vi "CRYMain Menu Process.vi"(3 "Sub Menu String":string, 4 "Menu String":string, 5 "nData":i32) -> (1 "sData_Out":string)   [LabVIEW 2013]
doc: "This is a subVI for the Block Menu Demo.vi. It is used as a pop-up subVI that displays a progress indicator."
uses:
  CRYProject/CRYProject Editor Global.vi
  CRYMainGlobal.vi
  DataView/VIEW/CRYView Global.vi
  DataView/VIEW/CRYNew View Global.vi
  CRYStepSetup/CRYStepSetup Global.vi
  CRYSystem/Task Sequence/CRYProject Run Control Global.vi
  SubVI/CRYMain Sub Window Global.vi
  CRYSystem/Data/CRYData & result stacks global.vi
  CRYSystem/Program/CRYRef nums global.vi
  CRYSystem/Misc/SubVI/CRYMisc vis settings global.vi
  <vilib>/Platform/browser.llb/Open URL in Default Browser (string).vi
  <vilib>/Platform/browser.llb/Open URL in Default Browser (path).vi
  <vilib>/Utility/miscctls.llb/LVRectTypeDef.ctl
panel:
  out "sData":string
  in  "pVIRef 2":refnum<vi>
  in  "pVIRef":refnum<vi>
  # "Main Menu Process"
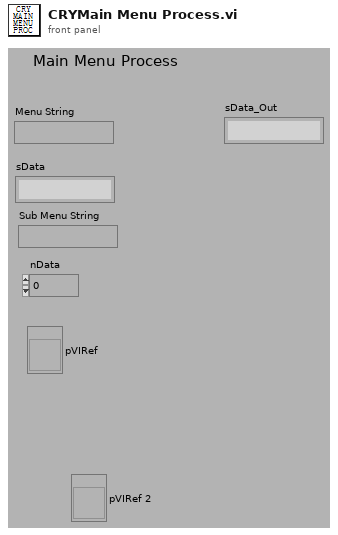
[diagram p1: front panel]
types:
  T1 = cluster{"EventName":string, "Arg1":string, "Numeric":u16, "Numeric 2":u16, "AddSteps ":refnum<vi>, "Arg1 2":string, "Arg1 3":string, "Boolean":bool}
  T2 = enum32{"Invalid", "Standard", "Closed", "Hidden", "Minimized", "Maximized"}
  T3 = enum16{"OK", "Yes", "YesNo", "YesNoCancel", "ReplaceAppend"}
  T4 = cluster{"sAction":string, "sType":string, "sQueueName":string, "sGraphName":string, "sData":string, "nData":i32, "pVIRef":refnum<vi>, "pSPRef":refnum<vi>}
  T5 = typedef "LVRectTypeDef.ctl" = cluster{"Left":i16, "Top":i16, "Right":i16, "Bottom":i16}
  T6 = typedef "CRYTS.ctl" = cluster{"No.TS":u16, "TS File Path":path, "TS Name":string, "EditStepName":string, "Steps":T7[], "New State":bool, "Change State":bool, "Flattened CurveLib Data":string, "Document Data":string, "EditStepNo":u16, "Operator Start File":string, "Sequence Type":string, "Sequence Language":string}
  T7 = typedef "CRYStep.ctl" = cluster{"No.VI":i32, "Category":string, "StepName":string, "Seq setup flattened":string, "Comment":string, "Steps config.":bool[], "Jump config":i32[], "Start":dbl, "Increment":dbl, "Name":string, "Unit":string, "Y data":u16, "Y prefix":string, "Y dB ref":dbl, "Y unit":string, "Repeat State Array":cluster{"Start":dbl, "Increment":dbl, "Count":i32, "Num":i32}[]}
  T8 = cluster{"nType":i32, "nParent":i32, "pVIW":refnum<vi>, "pSPW":refnum<vi>, "nTypeF":i32, "pVIF":refnum<vi>, "pSPF":refnum<vi>, "nIDSpliter":i32, "nProperty":i32, "Bound":T5, "nID":i32, "nData":i32, "sData":string, "pWVI":refnum<vi>, "sTitle":string, "cPages":cluster{"nPage":i32, "sTitle":string, "sIcon":string, "pVI":refnum<vi>, "nID":i32}[], "pTab":refnum<vi>, "nIDPages":i32[], "pSPT":refnum<vi>, "sTemp":string, "nDockID":i32, "nDockLR":i32, "sIcon":string}
  T9 = cluster{"nID":i32, "sName":string, "sType":string, "sProperty":string, "sTemplet":string, "sDocking":string, "pVIRef":refnum<vi>, "pSPRef":refnum<vi>, "pRefTemplet":refnum<vi>, "pRefSplitter":refnum<vi>[], "nPosSplitter":i32[], "pRefSP":refnum<vi>[], "nSPID":i32[], "sSPDock":string[], "nIDFrame":i32[], "nIDPanel":i32[], "nActiveFrame":i32, "nCountFrame":i32, "cFrame":cluster{"nID":i32, "sName":string, "sType":string, "sTitle":string, "sIcon":string, "pVIRef":refnum<vi>, "pSPRef":refnum<vi>, "cWiin":cluster{"sName":string, "sType":string, "pVIRef":refnum<vi>, "sData":string}, "cTab":cluster{"sTitle":string, "sIcon":string, "pSpliter":refnum<vi>, "nAvtivePage":i32, "nIDPage":i32[], "nIDFrame":i32[]}, "sData":string}[], "sData":string, "sSplitterName":string[]}
  T10 = cluster{"pw engr":string, "pw tech":string, "pw oper":string}
  T11 = enum32{"English", "Chinese", "Korean", "Japanese", "Russian", "Chinese traditional"}
  T12 = typedef "Graph Main Info Cluster.ctl" = cluster{"Selected_BarIdx":i32, "Selected_PanelIdx":i32, "Graph Main VIRef":refnum<vi>, "ToolBarClick":bool, "Spliter Ref Array":refnum<vi>[], "Panel Ref Array":refnum<vi>[], "Spliter_matrix":i32[][], "Panel_matrix":i32[][], "child_spliterIdx_matrix":i32[][], "split_pos_matrix":i32[][], "Title State":bool, "sQueueName":string, "Frame nID":i32, "Graph VIRef Array":cluster{"Graph VIRef":refnum<vi>, "Panel Idx":i32, "Frame VIRef":refnum<vi>, "Icon Ring":i32, "Graph Type":string}[], "View Type":string}
  T13 = cluster{"sStepName":string, "nStepVINo":i32, "nStepVINoDisplay":i32}
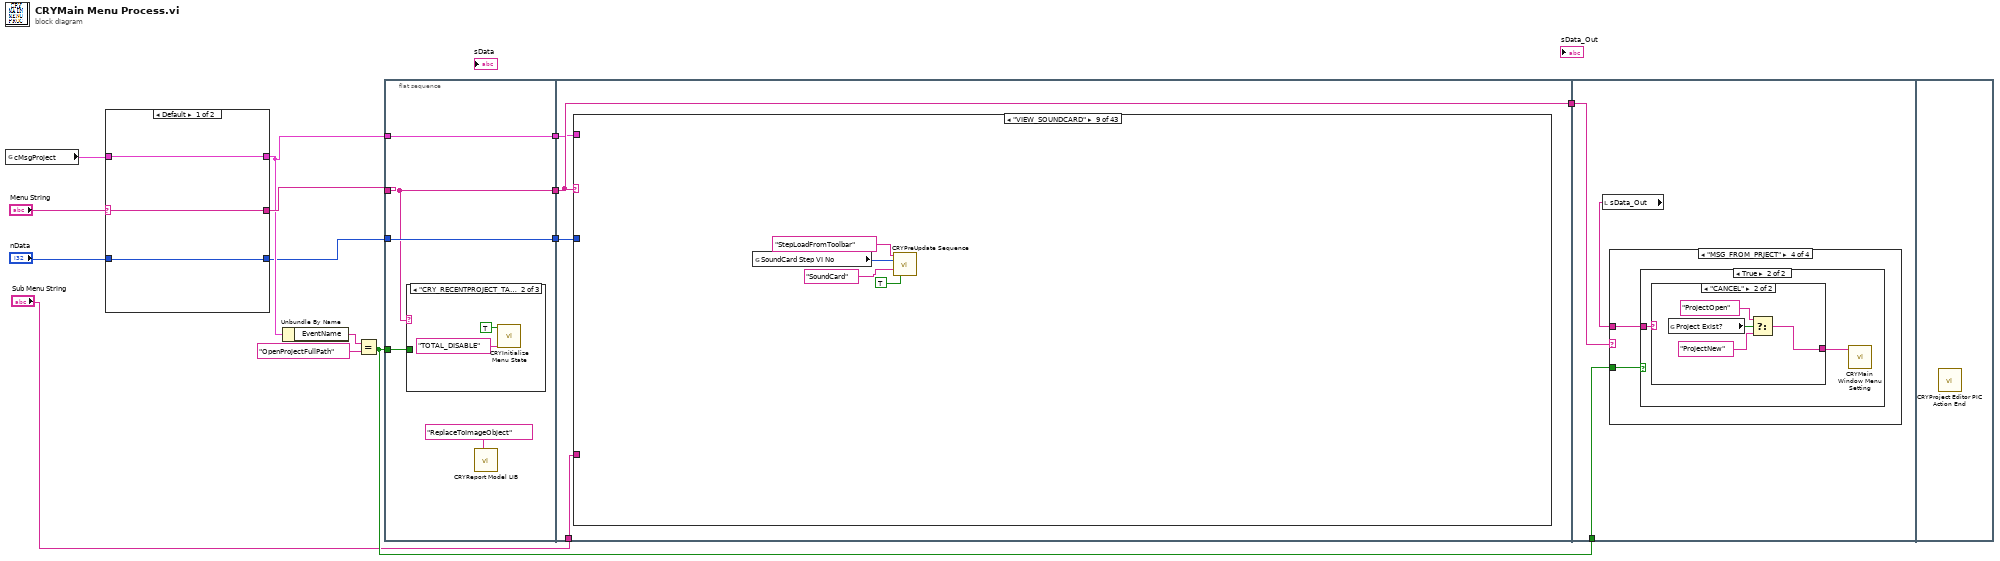
[diagram p0: block diagram]
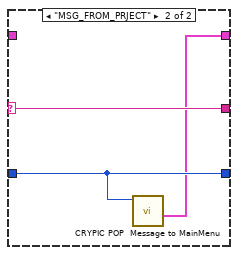
[diagram p2: hidden frame]
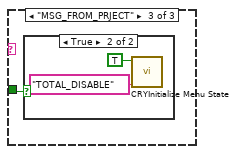
[diagram p4: hidden frame]
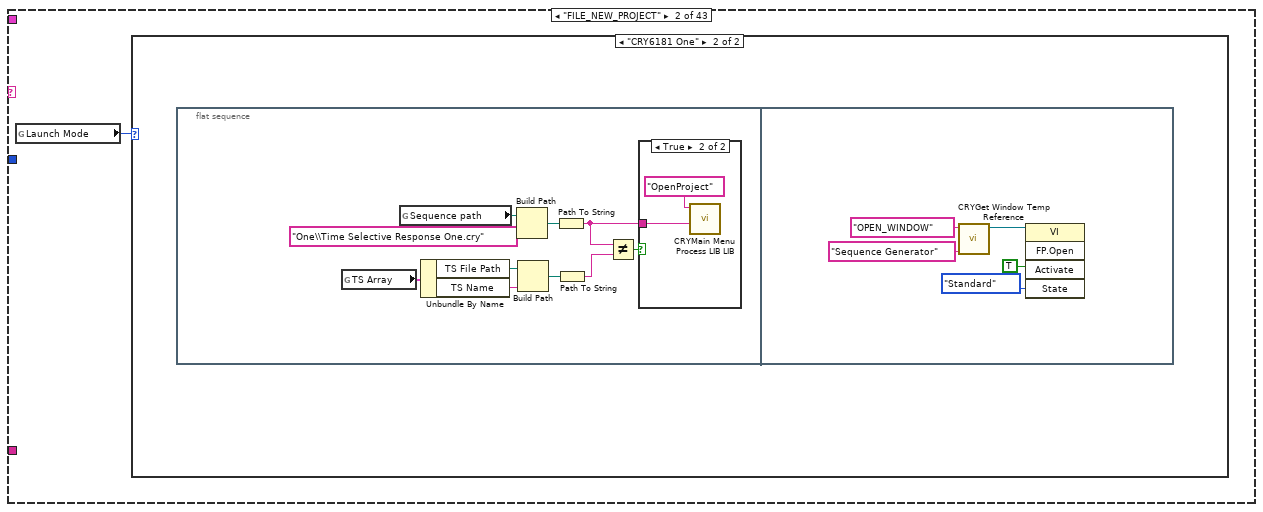
[diagram p7: hidden frame]
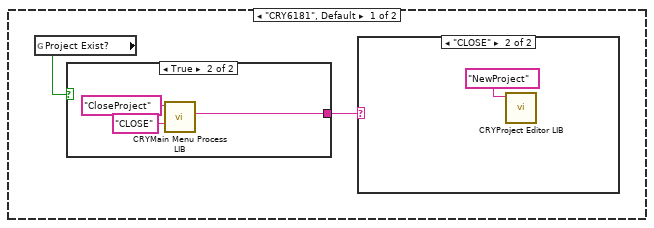
[diagram p8: hidden frame]
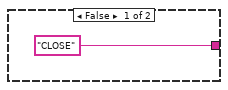
[diagram p10: hidden frame]
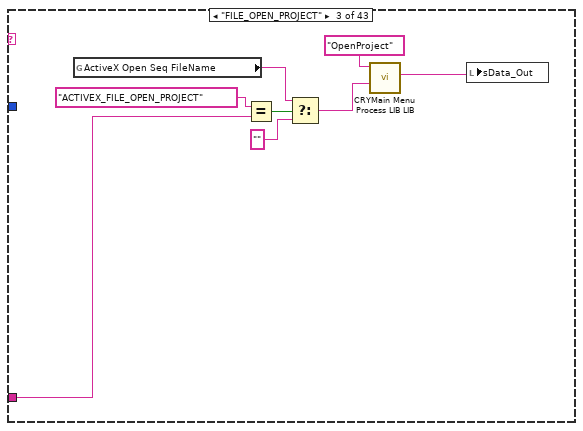
[diagram p12: hidden frame]
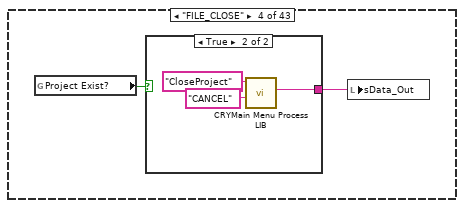
[diagram p13: hidden frame]
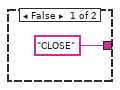
[diagram p14: hidden frame]
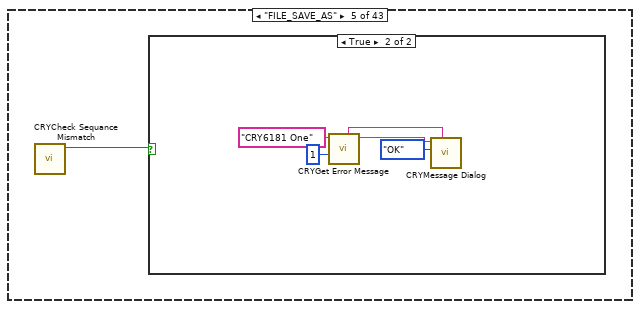
[diagram p15: hidden frame]
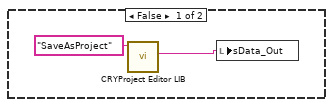
[diagram p16: hidden frame]
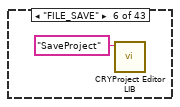
[diagram p17: hidden frame]
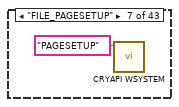
[diagram p18: hidden frame]
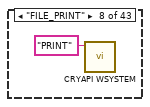
[diagram p19: hidden frame]
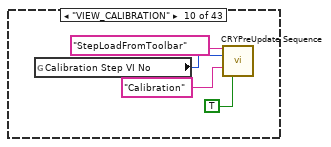
[diagram p20: hidden frame]
diagram:
  n1 = global read "CRYProject Editor Global.vi" "cMsgProject"() -> (w5:T1)
  n2 = case shown="Default" "Menu String" {
    selector: "Menu String" -> [w16 w20]
    tunnel: w5 -> [w17 _]
    tunnel: [w17 w18] -> w3
    tunnel: [w16 w20] -> w4
    tunnel: [w15 w19] -> w2
    tunnel: "nData" -> [w15 w19]
    frame Default {
    }
    frame "MSG_FROM_PRJECT" {
      n3 = call "CRYPIC POP  Message to MainMenu.vi"("nData"=w19) -> ("cMsgProject"=w18:T1)  [unwired: 10 in]
    }
  }
  n4 = Unbundle By Name(w3) -> ("EventName"=w10:string)
  n5 = Equal?(x=w10, y="OpenProjectFullPath" ("EventName")) -> (x = y?=w8:bool)
  n6 = flat-sequence {
    tunnel: w4 -> [w23]
    tunnel: [w23] -> w14
    tunnel: w2 -> [w24]
    tunnel: [w24] -> w13
    tunnel: [w22] -> w11
    tunnel: w3 -> [w22]
    tunnel: w8 -> [w21]
    tunnel: w14 -> [w33]
    tunnel: w13 -> [w34]
    tunnel: [w33] -> w12
    tunnel: w11 -> [w32]
    tunnel: "Sub Menu String" -> [w31]
    tunnel: w12 -> [w614]
    tunnel: w8 -> [w612]
    frame #0 {
      n7 = case shown="\"CRY_RECENTPROJECT_TAG0\", \"CRY_RECENTPROJECT_TAG1\", \"CRY_RECENTPROJECT_TAG2\", \"CRY_RECENTPROJECT_TAG3\", \"CRY_RECENTPROJECT_TAG4\", \"FILE_CLOSE\", \"FILE_NEW_PROJECT\", \"FILE_OPEN_PROJECT\", \"FILE_SAVE\", \"FILE_SAVE_AS\", \"MSG_OPEN_PROJECT\"" w23 {
        tunnel: w21 -> [_ _ w28]
        frame "False", Default {
        }
        frame "CRY_RECENTPROJECT_TAG0", "CRY_RECENTPROJECT_TAG1", "CRY_RECENTPROJECT_TAG2", "CRY_RECENTPROJECT_TAG3", "CRY_RECENTPROJECT_TAG4", "FILE_CLOSE", "FILE_NEW_PROJECT", "FILE_OPEN_PROJECT", "FILE_SAVE", "FILE_SAVE_AS", "MSG_OPEN_PROJECT" {
          n8 = call "CRYInitialize Menu State.vi"("sAction"="TOTAL_DISABLE", "Is Disable?"=TRUE) -> ()  [unwired: 10 in]
        }
        frame "MSG_FROM_PRJECT" {
          n9 = case shown="True" w28 {
            frame False {
            }
            frame True {
              n10 = call "CRYInitialize Menu State.vi"("sAction"="TOTAL_DISABLE", "Is Disable?"=TRUE) -> ()  [unwired: 10 in]
            }
          }
        }
      }
      n11 = call "CRYReport Model LIB.vi"("sAction"="ReplaceToImageObject") -> ()  [unwired: 9 in, 2 out]
    }
    frame #1 {
      n12 = case shown="\"VIEW_SOUNDCARD\"" w33 {
        selector: w33 -> [_ _ _ _ _ _ _ _ _ _ _ _ _ _ _ _ _ w187 w256 w267 _ w290 _ w294 _ _ _ _ _ _ _ _ _ _ w445 _ _ _ _ _ _ _ _]
        tunnel: w34 -> [_ _ _ _ _ _ _ _ _ _ _ _ _ _ _ _ _ _ _ _ _ _ _ _ _ _ _ _ _ _ _ _ _ _ _ _ w514 _ _ w568 _ _ _]
        tunnel: w32 -> [_ _ _ _ _ _ _ _ _ _ _ _ _ _ _ _ _ _ _ _ _ _ _ _ _ _ _ _ _ _ _ _ _ _ _ w453 _ _ _ _ _ _ _]
        tunnel: w31 -> [_ _ w61 _ _ _ _ _ _ _ _ _ _ _ _ _ _ _ _ _ _ _ _ _ _ _ _ _ _ _ _ _ _ _ _ _ _ _ _ _ _ _ _]
        frame Default {
        }
        frame "FILE_NEW_PROJECT" {
          n13 = global read "CRYMainGlobal.vi" "Launch Mode"() -> (w35:enum32{"CRY6181", "CRY6181 One"})
          n14 = case shown="\"CRY6181 One\"" w35 {
            frame "CRY6181", Default {
              n15 = global read "CRYProject Editor Global.vi" "Project Exist?"() -> (w37:bool)
              n16 = case shown="True" w37 {
                tunnel: ["CLOSE" ("sData_Out") w40] -> w36
                frame False {
                }
                frame True {
                  n17 = call "CRYMain Menu Process LIB.vi"("sOption"="CLOSE", "sAction"="CloseProject") -> ("sData_Out"=w40:string)  [unwired: 9 in]
                }
              }
              n18 = case shown="\"CLOSE\"" w36 {
                frame "CANCEL", Default {
                }
                frame "CLOSE" {
                  n19 = call "CRYProject Editor LIB.vi"("sAction"="NewProject") -> ()  [unwired: 10 in, 1 out]
                }
              }
            }
            frame "CRY6181 One" {
              n20 = flat-sequence {
                frame #0 {
                  n21 = global read "CRYProject Editor Global.vi" "TS Array"() -> (w49:T6)
                  n22 = global read "CRYMainGlobal.vi" "Sequence path"() -> (w50:path)
                  n23 = Unbundle By Name(w49) -> ("TS File Path"=w48:path, "TS Name"=w47:string)
                  n24 = Build Path(base path=w50, name or relative path="One\\Time Selective Response One.cry") -> (appended path=w51:path)
                  n25 = Build Path(base path=w48, name or relative path=w47) -> (appended path=w46:path)
                  n26 = Path To String(path=w51) -> (string=w45:string)
                  n27 = Path To String(path=w46) -> (string=w44:string)
                  n28 = Not Equal?(x=w45, y=w44) -> (x != y?=w43:bool)
                  n29 = case shown="True" w43 {
                    tunnel: w45 -> [_ w54]
                    frame False {
                    }
                    frame True {
                      n30 = call "CRYMain Menu Process LIB LIB.vi"("sOption"=w54, "sAction"="OpenProject") -> ()  [unwired: 9 in, 1 out]
                    }
                  }
                }
                frame #1 {
                  n31 = call "CRYGet Window Temp Reference.vi"("sWindowName"="Sequence Generator", "sAction"="OPEN_WINDOW") -> ("pVIRef_Out"=w55:refnum<vi>)  [unwired: 5 in, 4 out]
                  n32 = invoke class="VI" method="FP.Open"(reference=w55, "Activate"=TRUE ("Activate?"), "State"=T2."Standard") -> ()  [unwired: 2 in, 5 out]
                }
              }
            }
          }
        }
        frame "FILE_OPEN_PROJECT" {
          n33 = global read "CRYMainGlobal.vi" "ActiveX Open Seq FileName"() -> (w60:string)
          n34 = Equal?(x="ACTIVEX_FILE_OPEN_PROJECT" ("input 2"), y=w61) -> (x = y?=w65:bool)
          n35 = Select(t=w60, s=w65, f="" ("sOption")) -> (s? t:f=w63:string)
          n36 = call "CRYMain Menu Process LIB LIB.vi"("sOption"=w63, "sAction"="OpenProject") -> ("sData_Out"=w66:string)  [unwired: 9 in]
          n37 = local write "sData_Out"(w66) -> ()
        }
        frame "FILE_CLOSE" {
          n38 = global read "CRYProject Editor Global.vi" "Project Exist?"() -> (w69:bool)
          n39 = case shown="True" w69 {
            tunnel: ["CLOSE" ("sData_Out") w71] -> w68
            frame False {
            }
            frame True {
              n40 = call "CRYMain Menu Process LIB.vi"("sOption"="CANCEL", "sAction"="CloseProject") -> ("sData_Out"=w71:string)  [unwired: 9 in]
            }
          }
          n41 = local write "sData_Out"(w68) -> ()
        }
        frame "FILE_SAVE_AS" {
          n42 = call "CRYCheck Sequance Mismatch.vi"() -> ("Mismatch"=w74:bool)  [unwired: 10 in, 1 out]
          n43 = case shown="True" w74 {
            frame False {
              n44 = call "CRYProject Editor LIB.vi"("sAction"="SaveAsProject") -> ("sData_Out"=w75:string)  [unwired: 10 in]
              n45 = local write "sData_Out"(w75) -> ()
            }
            frame True {
              n46 = call "CRYGet Error Message.vi"("Error No"=1, "Kind"="CRY6181 One") -> ("Message"=w80:string, "Window Title"=w79:string)  [unwired: 4 in, 4 out]
              n47 = call "CRYMessage Dialog.vi"("Window Title"=w79, "YesNoCancel"=T3."OK", "Message Content"=w80) -> ()  [unwired: 7 in, 2 out]
            }
          }
        }
        frame "FILE_SAVE" {
          n48 = call "CRYProject Editor LIB.vi"("sAction"="SaveProject") -> ()  [unwired: 10 in, 1 out]
        }
        frame "FILE_PAGESETUP" {
          n49 = call "CRYAPI WSYSTEM.vi"("sAction"="PAGESETUP") -> ()  [unwired: 7 in, 4 out]
        }
        frame "FILE_PRINT" {
          n50 = call "CRYAPI WSYSTEM.vi"("sAction"="PRINT") -> ()  [unwired: 7 in, 4 out]
        }
        frame "VIEW_SOUNDCARD" {
          n51 = global read "CRYProject Editor Global.vi" "SoundCard Step VI No"() -> (w88:i32)
          n52 = call "CRYPreUpdate Sequence.vi"("EventName"="StepLoadFromToolbar", "Proper VI No"=w88, "Project View Step Name Identifier Arg1"="SoundCard", "AllChangeFlg"=TRUE) -> ()  [unwired: 12 in]
        }
        frame "VIEW_CALIBRATION" {
          n53 = global read "CRYProject Editor Global.vi" "Calibration Step VI No"() -> (w92:i32)
          n54 = call "CRYPreUpdate Sequence.vi"("EventName"="StepLoadFromToolbar", "Proper VI No"=w92, "Project View Step Name Identifier Arg1"="Calibration", "AllChangeFlg"=TRUE) -> ()  [unwired: 12 in]
        }
        frame "VIEW_DATA_VIEW" {
          n55 = flat-sequence {
            frame #0 {
              n56 = call "CRYSet Drop Data.vi"("Graph Type In"="XY" ("DataType In")) -> ()  [unwired: 11 out]
            }
            frame #1 {
              n57 = call "CRYAPI WSYSTEM.vi"("sData"="DataView" ("Window Type"), "sAction"="DOCK_TAB") -> ()  [unwired: 2 in, 8 out]
            }
          }
        }
        frame "VIEW_DATA_VIEW_TEMPLATE" {
          n58 = flat-sequence {
            tunnel: [w106] -> w100
            tunnel: [w105] -> w99
            tunnel: [w104] -> w98
            tunnel: [w101] -> w97
            tunnel: w100 -> [w120]
            tunnel: w99 -> [w119]
            tunnel: w98 -> [w118]
            tunnel: w97 -> [w117]
            tunnel: [w116] -> w96
            tunnel: w96 -> [w158]
            frame #0 {
              n59 = call "CRYAPI WSYSTEM.vi"("sData"="DataView" ("Window Type"), "sAction"="DOCK_TAB") -> ("tFrame_Out"=w107:T8)  [unwired: 2 in, 7 out]
              n60 = Unbundle By Name(w107) -> ("pWVI"=w103:refnum<vi>)
              n61 = Not A Number/Path/Refnum?(number/path/refnum=w103) -> (NaN/Path/Refnum?=w102:bool)
              n62 = Not(x=w102) -> (.not. x?=w101:bool)
              n63 = case shown="False" w101 {
                tunnel: [_ w115] -> w106
                tunnel: [_ w114] -> w105
                tunnel: [_ w113] -> w104
                tunnel: w103 -> [_ w110]
                frame False {
                }
                frame True {
                  n64 = invoke class="VI" method="Ctrl Val.Get"(reference=w110, "Control Name"="nIDV") -> (reference out=w113:refnum<vi>, "Get Control Value Variant"=w114:variant)  [unwired: 2 in, 2 out]
                  n65 = invoke class="VI" method="Ctrl Val.Get"(reference=w110, "Control Name"="cNewBootVIEW") -> ("Get Control Value Variant"=w115:variant)  [unwired: 2 in, 3 out]
                }
              }
            }
            frame #1 {
              n66 = case shown="True" w117 {
                tunnel: w120 -> [_ w125]
                tunnel: w119 -> [_ w124]
                tunnel: w118 -> [_ w123]
                tunnel: [-1 ("nID") w122] -> w116
                frame False {
                }
                frame True {
                  n67 = global read "CRYMainGlobal.vi" "Steps path"() -> (w131:path)
                  n68 = Build Path(base path=w131, name or relative path="CRYDisplay") -> (appended path=w130:path)
                  n69 = Build Path(base path=w130, name or relative path="align_template.dis") -> (appended path=w128:path)
                  n70 = Read from Binary File(10:-1 ("count (1)"), 11:w128) -> (2:w126:string)  [unwired: 4 in, 3 out]
                  n71 = call "CRYDataView Pic LIB.vi"("sAction"="CheckData", "sOption"=w126) -> ("nData_Out"=w133:i32)  [unwired: 7 in, 2 out]
                  n72 = case shown="Default" w133 {
                    tunnel: w126 -> [_ w148]
                    tunnel: w125 -> [_ w145]
                    tunnel: w124 -> [_ w142]
                    tunnel: w123 -> [_ w139]
                    tunnel: [-1 ("nID") w136] -> w122
                    frame -1 {
                    }
                    frame Default {
                      n73 = flat-sequence {
                        tunnel: w146 -> [w152]
                        tunnel: w139 -> [w153]
                        tunnel: [w150] -> w138
                        tunnel: w138 -> [w157]
                        frame #0 {
                          n74 = invoke class="VI" method="Ctrl Val.Set"(reference=w153, "Control Name"="pGraphMain VI Ref", "Value"=w152) -> (reference out=w150:refnum<vi>)  [unwired: 2 in, 4 out]
                        }
                        frame #1 {
                          n75 = call "CRYGet Boolean Reference.vi"("Label Name"="AttachView", "VI Refnum"=w157) -> ("Boolean Ref"=w155:refnum<vi>)  [unwired: 7 in, 2 out]
                          n76 = property class="Bool"(reference=w155, "Val(Sgnl)"=TRUE ("Value (Signaling)")) -> ()  [unwired: 1 in, 2 out]
                        }
                      }
                      n77 = Variant To Data(type=T4 {"sAction"="", "sType"="", "sQueueName"="", "sGraphName"="", "sData"="", "nData"=0, "pVIRef"=refnum, "pSPRef"=refnum} ("cNewBootVIEW"), Variant=w145) -> (data=w143:T4)  [unwired: 1 in, 1 out]
                      n78 = Variant To Data(type=0, Variant=w142) -> (data=w140:i32)  [unwired: 1 in, 1 out]
                      n79 = call "CRYDataView Function LIB.vi"("sAction"="LoadView", "nData"=w140, "sData"=w148, "cBootVIEW"=w143) -> ("cView_Out"=w147:T9)  [unwired: 5 in, 2 out]
                      n80 = Unbundle By Name(w147) -> ("pVIRef"=w146:refnum<vi>, "nID"=w136:i32, "sName"=w137:string)
                      n81 = global write "CRYView Global.vi" "sActiveView"(w137) -> ()
                    }
                  }
                }
              }
            }
            frame #2 {
              n82 = case shown="Default" w158 {
                selector: w158 -> [_ w161]
                frame -1 {
                }
                frame Default {
                  n83 = call "CRYView Out CurLibrary.vi"("DataView Idx"=w161, "sData"="GRAPH_TITLE_CLICK", "sAction"="WinActive") -> ()  [unwired: 7 in, 2 out]
                }
              }
              n84 = global write "CRYNew View Global.vi" "g_WaitFlag"(FALSE ("g_WaitFlag")) -> ()
            }
          }
        }
        frame "VIEW_STEP_SETUP" {
          n85 = call "CRYCheck Sequance Mismatch.vi"() -> ("Match"=w163:bool)  [unwired: 10 in, 1 out]
          n86 = case shown="True" w163 {
            frame False {
              n87 = call "CRYAPI WSYSTEM.vi"("sData"="Step Setup" ("Window Type"), "sAction"="DOCK_TAB") -> ()  [unwired: 2 in, 8 out]
            }
            frame True {
              n88 = flat-sequence {
                frame #0 {
                  n89 = global write "CRYStepSetup Global.vi" "Step Setup Clicked"(TRUE ("Step Step Clicked")) -> ()
                }
                frame #1 {
                  n90 = call "CRYGet Window Temp Reference.vi"("sWindowName"="Sequence Generator", "sAction"="OPEN_WINDOW") -> ("pVIRef_Out"=w167:refnum<vi>)  [unwired: 5 in, 4 out]
                  n91 = invoke class="VI" method="FP.Open"(reference=w167, "Activate"=TRUE ("Activate?"), "State"=T2."Standard") -> ()  [unwired: 2 in, 5 out]
                }
              }
            }
          }
        }
        frame "VIEW_DOCUMENT" {
          n92 = call "CRYReport Check.vi"() -> ("bResult"=w172:bool)  [unwired: 11 in]
          n93 = case shown="False" w172 {
            frame False {
              n94 = call "CRYGet Error Message.vi"("Error No"=1, "Kind"="Document") -> ("Message"=w177:string, "Window Title"=w176:string)  [unwired: 4 in, 4 out]
              n95 = call "CRYMessage Dialog.vi"("Window Title"=w176, "YesNoCancel"=T3."OK", "Message Content"=w177) -> ()  [unwired: 7 in, 2 out]
            }
            frame True {
              n96 = call "CRYAPI WSYSTEM.vi"("sData"="Document" ("Window Type"), "sAction"="DOCK_TAB") -> ()  [unwired: 2 in, 8 out]
            }
          }
        }
        frame "VIEW_CURVES_LIBRARY" {
          n97 = call "CRYAPI WSYSTEM.vi"("sData"="Curves Library" ("Window Type"), "sAction"="DOCK_LEFT_WIN") -> ()  [unwired: 2 in, 8 out]
        }
        frame "VIEW_PROJECT" {
          # "Window Open State Find ???????????"
          n98 = call "CRYAPI WSYSTEM.vi"("sData"="Project" ("Window Type"), "sAction"="DOCK_LEFT_WIN") -> ()  [unwired: 2 in, 8 out]
        }
        frame "VIEW_RESULT" {
          # "Window Open State Find ???????????"
          n99 = flat-sequence {
            frame #0 {
              n100 = call "CRYSet Drop Data.vi"("Graph Type In"="WAVE" ("DataType In")) -> ()  [unwired: 11 out]
            }
            frame #1 {
              n101 = call "CRYAPI WSYSTEM.vi"("sData"="Result View" ("Window Type"), "sAction"="DOCK_TAB") -> ()  [unwired: 2 in, 8 out]
            }
          }
        }
        frame "TOOLS_CONTINUE", "TOOLS_REDO", "TOOLS_START" {
          n102 = global read "CRYProject Run Control Global.vi" "RunState"() -> (w188:bool)
          n103 = case shown="False" w188 {
            tunnel: w187 -> [w190 _]
            frame False {
              n104 = call "CRYLicense Manager.vi"() -> ("Test Result"=w189:bool)  [unwired: 10 in, 1 out]
              n105 = case shown="True" w189 {
                tunnel: w190 -> [_ w207]
                frame False {
                  n106 = flat-sequence {
                    frame #0 {
                      n107 = call "CRYGet Error Message.vi"("Error No"=26, "Kind"="Project") -> ("Message"=w194:string, "Window Title"=w193:string)  [unwired: 4 in, 4 out]
                      n108 = call "CRYMessage Dialog.vi"("Window Title"=w193, "YesNoCancel"=T3."OK", "Message Content"=w194) -> ()  [unwired: 7 in, 2 out]
                    }
                    frame #1 {
                      n109 = global read "CRYMain Sub Window Global.vi" "Main VI Ref"() -> (w196:refnum<vi>)
                      n110 = call "CRYGet Boolean Reference.vi"("Label Name"="Start", "VI Refnum"=w196) -> ("Boolean Ref"=w204:refnum<vi>)  [unwired: 7 in, 2 out]
                      n111 = call "CRYGet Boolean Reference.vi"("Label Name"="Redo", "VI Refnum"=w196) -> ("Boolean Ref"=w202:refnum<vi>)  [unwired: 7 in, 2 out]
                      n112 = call "CRYGet Boolean Reference.vi"("Label Name"="Continue", "VI Refnum"=w196) -> ("Boolean Ref"=w197:refnum<vi>)  [unwired: 7 in, 2 out]
                      n113 = property class="Bool"(reference=w202, "Value"=FALSE) -> ()  [unwired: 1 in, 2 out]
                      n114 = property class="Bool"(reference=w197, "Value"=FALSE) -> ()  [unwired: 1 in, 2 out]
                      n115 = property class="Bool"(reference=w204, "Value"=FALSE) -> ()  [unwired: 1 in, 2 out]
                    }
                  }
                }
                frame True {
                  n116 = call "CRYCheck Sequance Mismatch.vi"() -> ("Mismatch"=w206:bool)  [unwired: 10 in, 1 out]
                  n117 = case shown="False" w206 {
                    tunnel: w207 -> [w210 _]
                    frame False {
                      n118 = case shown="\"TOOLS_REDO\"" w210 {
                        tunnel: [FALSE ("Redo") TRUE ("Redo")] -> w209
                        frame Default {
                        }
                        frame "TOOLS_REDO" {
                        }
                      }
                      n119 = disable-structure shown="Enabled" {
                        disable-tunnel: w209 -> [_ _]
                        frame Disabled {
                          n120 = global read "CRYRef nums global.vi" "Run project VI ref"() -> (w225:refnum<vi>)
                          n121 = global read "CRYMain Sub Window Global.vi" "Main VI Ref"() -> (w232:refnum<vi>)
                          n122 = property class="VI"(reference=w225) -> (reference out=w224:refnum<vi>, error out=w218:errorcluster, "Front Panel.PanelBounds"=w217:T5)  [unwired: 1 in]
                          n123 = property class="VI"(reference=w232) -> ("Front Panel.PanelBounds"=w231:T5)  [unwired: 1 in, 2 out]
                          n124 = Unbundle By Name(w217) -> ("Right"=w216:i16, "Left"=w215:i16, "Bottom"=w214:i16, "Top"=w213:i16)
                          n125 = Unbundle By Name(w231) -> ("Left"=w230:i16, "Bottom"=w228:i16)
                          n126 = Subtract(x=w216, y=w215) -> (x-y=w212:i16)
                          n127 = Subtract(x=w214, y=w213) -> (x-y=w211:i16)
                          n128 = Add(x=w230, y=w212) -> (x+y=w229:i16)
                          n129 = Subtract(x=w228, y=w211) -> (x-y=w227:i16)
                          n130 = Bundle By Name(cluster=T5 {"Left"=0, "Top"=0, "Right"=0, "Bottom"=0} ("Front Panel Window:Panel Bounds"), "Left"=w230, "Bottom"=w228, "Right"=w229, "Top"=w227) -> (w219:T5)
                          n131 = invoke class="VI" method="Run VI"(reference=w224, error in=w218, "Wait until done"=FALSE ("Wait Until Done")) -> (reference out=w223:refnum<vi>, error out=w221:errorcluster)  [unwired: 2 in, 3 out]
                          n132 = property class="VI"(reference=w223, error in=w221, "Front Panel.PanelBounds"=w219) -> (reference out=w222:refnum<vi>, error out=w220:errorcluster)
                          n133 = property class="VI"(reference=w222, error in=w220, "Front Panel.Open"=TRUE ("Front Panel Window:Open")) -> ()  [unwired: 2 out]
                        }
                        frame Enabled {
                          n134 = global read "CRYRef nums global.vi" "Run project VI ref"() -> (w235:refnum<vi>)
                          n135 = invoke class="VI" method="Run VI"(reference=w235, "Wait until done"=FALSE ("Wait Until Done")) -> ()  [unwired: 3 in, 5 out]
                        }
                      }
                      n136 = case shown="\"TOOLS_CONTINUE\"" w210 {
                        frame Default {
                        }
                        frame "TOOLS_CONTINUE" {
                          n137 = global write "CRYProject Run Control Global.vi" "Cont State"(TRUE ("Cont State")) -> ()
                        }
                      }
                      n138 = global write "CRYData & result stacks global.vi" "Redo"(w209) -> ()
                      n139 = call "CRYStep Save Close.vi"("sAction"="SaveClose") -> ()  [unwired: 11 in]
                    }
                    frame True {
                      n140 = flat-sequence {
                        frame #0 {
                          n141 = call "CRYGet Error Message.vi"("Error No"=0, "Kind"="CRY6181 One") -> ("Message"=w243:string, "Window Title"=w242:string)  [unwired: 4 in, 4 out]
                          n142 = call "CRYMessage Dialog.vi"("Window Title"=w242, "YesNoCancel"=T3."OK", "Message Content"=w243) -> ()  [unwired: 7 in, 2 out]
                        }
                        frame #1 {
                          n143 = global read "CRYMain Sub Window Global.vi" "Main VI Ref"() -> (w245:refnum<vi>)
                          n144 = call "CRYGet Boolean Reference.vi"("Label Name"="Start", "VI Refnum"=w245) -> ("Boolean Ref"=w253:refnum<vi>)  [unwired: 7 in, 2 out]
                          n145 = call "CRYGet Boolean Reference.vi"("Label Name"="Redo", "VI Refnum"=w245) -> ("Boolean Ref"=w251:refnum<vi>)  [unwired: 7 in, 2 out]
                          n146 = call "CRYGet Boolean Reference.vi"("Label Name"="Continue", "VI Refnum"=w245) -> ("Boolean Ref"=w246:refnum<vi>)  [unwired: 7 in, 2 out]
                          n147 = property class="Bool"(reference=w251, "Value"=FALSE) -> ()  [unwired: 1 in, 2 out]
                          n148 = property class="Bool"(reference=w246, "Value"=FALSE) -> ()  [unwired: 1 in, 2 out]
                          n149 = property class="Bool"(reference=w253, "Value"=FALSE) -> ()  [unwired: 1 in, 2 out]
                        }
                      }
                    }
                  }
                }
              }
            }
            frame True {
            }
          }
        }
        frame "TOOLS_CONTINUE_STOP", "TOOLS_STOP" {
          n150 = case shown="False" FALSE {
            tunnel: w256 -> [w257 _]
            frame False {
              n151 = case shown="\"TOOLS_CONTINUE_STOP\"" w257 {
                frame Default {
                  n152 = global read "CRYMainGlobal.vi" "Seq Abort Ref"() -> (w259:refnum<vi>)
                  n153 = global write "CRYProject Run Control Global.vi" "Aborted"(TRUE ("StartState")) -> ()
                  n154 = property class="Bool (strict)"(reference=w259, "Val(Sgnl)"=TRUE ("Value (Signaling)")) -> ()  [unwired: 1 in, 2 out]
                }
                frame "TOOLS_CONTINUE_STOP" {
                  n155 = global read "CRYProject Run Control Global.vi" "RunState"() -> (w261:bool)
                  n156 = case shown="True" w261 {
                    frame False {
                    }
                    frame True {
                      n157 = global read "CRYProject Run Control Global.vi" "Cont State"() -> (w265:bool)
                      n158 = global read "CRYMainGlobal.vi" "Seq Abort Ref"() -> (w263:refnum<vi>)
                      n159 = Not(x=w265) -> (.not. x?=w264:bool)
                      n160 = property class="Bool (strict)"(reference=w263, "Val(Sgnl)"=TRUE ("Value (Signaling)")) -> ()  [unwired: 1 in, 2 out]
                      n161 = global write "CRYProject Run Control Global.vi" "Cont State"(w264) -> ()
                    }
                  }
                }
              }
            }
            frame True {
            }
          }
        }
        frame "OPERATOR_MULTIMETER", "OPERATOR_OSCILLOSCOPE", "OPERATOR_RTA", "OPERATOR_SIGGEN", "OPERATOR_SPECTRUM" {
          n162 = call "CRYOperator Process.vi"("sAction"="Open", "sOperator Type"=w267) -> ()  [unwired: 9 in, 1 out]
        }
        frame "OPERATOR_OPEN_CONFIGURATION" {
          n163 = call "CRYLoad Operator Window Configure.vi"() -> ("error out"=w271:errorcluster, "ok status"=w269:bool, "Flatten Step"=w270:string, "selected path"=w268:path)  [unwired: 8 in]
          n164 = case shown="No Error" w271 {
            tunnel: w270 -> [w273 _]
            tunnel: w269 -> [w274 w285]
            tunnel: w268 -> [w272 _]
            frame No Error {
              n165 = case shown="True" w274 {
                tunnel: w273 -> [_ w278]
                tunnel: w272 -> [_ w275]
                frame False {
                }
                frame True {
                  n166 = flat-sequence {
                    tunnel: [w280] -> w277
                    tunnel: w278 -> [w280]
                    tunnel: [w279] -> w276
                    tunnel: w275 -> [w279]
                    tunnel: w277 -> [w284]
                    tunnel: w276 -> [w282]
                    frame #0 {
                      n167 = call "CRYOperator Process.vi"("sAction"="RunCloseAll") -> ()  [unwired: 10 in, 1 out]
                    }
                    frame #1 {
                      n168 = call "CRYOperator Process.vi"("sAction"="OpenAll", "sOperator Type"=w284) -> ()  [unwired: 9 in, 1 out]
                      n169 = global write "CRYMisc vis settings global.vi" "Operator Work Path"(w282) -> ()
                    }
                  }
                }
              }
            }
            frame Error {
              n170 = case shown="True" w285 {
                frame False {
                }
                frame True {
                  n171 = call "CRYGet Error Message.vi"("Error No"=1, "Kind"="Operator Configure") -> ("Message"=w289:string, "Window Title"=w288:string)  [unwired: 4 in, 4 out]
                  n172 = call "CRYMessage Dialog.vi"("Window Title"=w288, "Message Content"=w289) -> ()  [unwired: 8 in, 2 out]
                }
              }
            }
          }
        }
        frame "OPERATOR_SAVEAS_CONFIGURATION", "OPERATOR_SAVE_CONFIGURATION" {
          n173 = call "CRYSave Operator Window Configure.vi"("Save Mode"=w290) -> ()  [unwired: 10 in, 1 out]
        }
        frame "OPERATOR_STARTUP_CONFIGURATION" {
          n174 = call "CRYSelect Operator Window Configure.vi"() -> ()  [unwired: 9 in, 3 out]
        }
        frame "CRY_RECENTOPERATOR_TAG0", "CRY_RECENTOPERATOR_TAG1", "CRY_RECENTOPERATOR_TAG2", "CRY_RECENTOPERATOR_TAG3", "CRY_RECENTOPERATOR_TAG4" {
          n175 = Match Pattern(string=w294, regular expression="_TAG") -> (after substring=w291:string)  [unwired: 1 in, 3 out]
          n176 = String Length(string=w291) -> (length=w292:i32)
          n177 = case shown="Default" w292 {
            tunnel: w291 -> [w304 _]
            frame Default {
              n178 = global read "CRYMainGlobal.vi" "Recent Item Names"() -> (w303:string[][])
              n179 = Decimal String To Number(string=w304) -> (number=w295:i32)  [unwired: 2 in, 1 out]
              n180 = Index Array(array=w303, index (row)=1 ("disabled index (col)"), index (col)=w295) -> (element=w298:string)
              n181 = String To Path(string=w298) -> (path=w297:path)
              n182 = call "CRYLoad Operator Window Configure.vi"("File path"=w297) -> ("error out"=w302:errorcluster, "ok status"=w300:bool, "Flatten Step"=w301:string, "selected path"=w299:path)  [unwired: 7 in]
              n183 = case shown="No Error" w302 {
                tunnel: w301 -> [w306 _]
                tunnel: w300 -> [w307 w318]
                tunnel: w299 -> [w305 _]
                frame No Error {
                  n184 = case shown="True" w307 {
                    tunnel: w306 -> [_ w311]
                    tunnel: w305 -> [_ w308]
                    frame False {
                    }
                    frame True {
                      n185 = flat-sequence {
                        tunnel: [w313] -> w310
                        tunnel: w311 -> [w313]
                        tunnel: [w312] -> w309
                        tunnel: w308 -> [w312]
                        tunnel: w310 -> [w317]
                        tunnel: w309 -> [w315]
                        frame #0 {
                          n186 = call "CRYOperator Process.vi"("sAction"="RecentRunCloseAll") -> ()  [unwired: 10 in, 1 out]
                        }
                        frame #1 {
                          n187 = call "CRYOperator Process.vi"("sAction"="OpenAll", "sOperator Type"=w317) -> ()  [unwired: 9 in, 1 out]
                          n188 = global write "CRYMisc vis settings global.vi" "Operator Work Path"(w315) -> ()
                        }
                      }
                    }
                  }
                }
                frame Error {
                  n189 = case shown="True" w318 {
                    frame False {
                    }
                    frame True {
                      n190 = call "CRYGet Error Message.vi"("Error No"=1, "Kind"="Operator Configure") -> ("Message"=w322:string, "Window Title"=w321:string)  [unwired: 4 in, 4 out]
                      n191 = call "CRYMessage Dialog.vi"("Window Title"=w321, "Message Content"=w322) -> ()  [unwired: 8 in, 2 out]
                    }
                  }
                }
              }
            }
            frame 0 {
            }
          }
        }
        frame "OPERATOR_CLOSEALL" {
          n192 = call "CRYOperator Process.vi"("sAction"="RunCloseAll") -> ()  [unwired: 10 in, 1 out]
        }
        frame "TOOLS_LOTPAUSE" {
          n193 = call "CRYInit Data & result stacks global.vi"("No Project Exist?"=FALSE ("New?"), "Pause Proc"=TRUE ("Pause"), "Init?"=FALSE) -> ()  [unwired: 9 in]
        }
        frame "TOOLS_CHANGE_PASSWORD" {
          n194 = flat-sequence {
            frame #0 {
              n195 = global write "CRYMainGlobal.vi" "Login Exit"(FALSE ("Login Exit")) -> ()
            }
            frame #1 {
              n196 = global read "CRYMainGlobal.vi" "Login vi path"() -> (w328:path)
              n197 = Open VI Reference(vi path=w328) -> (vi reference=w334:refnum<vi>, error out=w330:errorcluster)  [unwired: 1 in, 4 out]
              n198 = call "CRYGet Window Title Message.vi"("No"=7, "Kind"="Main") -> ("Multibyte String"=w337:string)  [unwired: 4 in, 5 out]
              n199 = call "CRYSet Login Front Panel.vi"("Vi Ref in"=w334) -> ("Vi Ref out"=w338:refnum<vi>)  [unwired: 10 in]
              n200 = property class="VI"(reference=w338, "Front Panel.Title"=w337) -> (reference out=w339:refnum<vi>)  [unwired: 1 in, 1 out]
              n201 = invoke class="VI" method="Run VI"(reference=w339, error in=w330, "Wait until done"=FALSE) -> (reference out=w332:refnum<vi>, error out=w333:errorcluster)  [unwired: 2 in, 3 out]
              n202 = property class="VI"(reference=w332, error in=w333, "Front Panel Window:Open"=TRUE ("Front Panel.Open")) -> ()  [unwired: 2 out]
            }
            frame #2 {
              n203 = while {
                stop <- w341 stop-if-true
                n204 = global read "CRYMainGlobal.vi" "Login Exit"() -> (w341:bool)
                n205 = Wait (ms)(milliseconds to wait=u32 10) -> ()  [unwired: 1 out]
              }
            }
            frame #3 {
              n206 = global read "CRYMainGlobal.vi" "Login State"() -> (w342:bool)
              n207 = case shown="False" w342 {
                frame False {
                  n208 = call "CRYInitialize Menu State.vi"() -> ()  [unwired: 12 in]
                  n209 = call "CRYUpdate State by User Level.vi"() -> ()  [unwired: 12 in]
                }
                frame True {
                }
              }
            }
          }
          n210 = disable-structure shown="Disabled" {
            frame Disabled {
              n211 = call "CRYLogin Read Config.vi"() -> ("Remember Out"=w350:bool, "Password out"=w349:T10, "Level Out"=w348:i32, "Login Section Out"=w351:cluster{"Key":string, "Value":string}[])  [unwired: 8 in]
              n212 = call "CRYLogin setup.vi"("Ask"=w350) -> ("Cancelled?"=w345:bool, "New PW?"=w346:bool, "Password"=w347:string)  [unwired: 5 in, 1 out]
              n213 = case shown="False" w345 {
                tunnel: w347 -> [w353 _]
                tunnel: w348 -> [w356 _]
                tunnel: [w355 w371] -> w344
                tunnel: w349 -> [w354 w371]
                tunnel: w346 -> [w352 _]
                frame False {
                  n214 = case shown="True" w352 {
                    tunnel: w353 -> [_ w359]
                    tunnel: w354 -> [w357 w358]
                    tunnel: [w357 w361] -> w355
                    tunnel: w356 -> [_ w360]
                    frame False {
                    }
                    frame True {
                      n215 = case shown="2.." w360 {
                        tunnel: w359 -> [w363 w366 w370]
                        tunnel: [w364 w367 w369] -> w361
                        tunnel: w358 -> [w362 w365 w368]
                        frame ..0 {
                          n216 = Bundle By Name(cluster=w362, "pw engr"=w363) -> (w364:T10)
                        }
                        frame 1 {
                          n217 = Bundle By Name(cluster=w365, "pw tech"=w366) -> (w367:T10)
                        }
                        frame 2.. {
                          n218 = Bundle By Name(cluster=w368, "pw oper"=w370) -> (w369:T10)
                        }
                      }
                    }
                  }
                }
                frame True {
                }
              }
              n219 = global read "CRYMainGlobal.vi" "user name"() -> (w343:string)
              n220 = call "CRYLogin Write Config.vi"("User Name In"=w343, "Remember In"=w350, "Password  In"=w344, "Level In"=w348, "Login Section In"=w351) -> ()  [unwired: 7 in]
            }
            frame Enabled {
            }
          }
        }
        frame "TOOLS_OPTION" {
          n221 = call "CRYOption Setting.vi"() -> ("Language Mode Change"=w372:bool, "Launch Mode Change"=w373:bool, "OK Flag"=w376:bool)  [unwired: 9 in]
          n222 = Or(x=w373, y=w372) -> (x .or. y?=w374:bool)
          n223 = Compound Arithmetic op=AND(w376, w374) -> (w375:bool)
          n224 = case shown="True" w375 {
            tunnel: w373 -> [_ w377]
            frame False {
            }
            frame True {
              n225 = flat-sequence {
                tunnel: w377 -> [w381]
                frame #0 {
                  n226 = Select(t=9 ("Error No"), s=w381, f=10) -> (s? t:f=w378:i32)
                  n227 = call "CRYGet Error Message.vi"("Error No"=w378, "Kind"="Main") -> ("Message"=w383:string, "Window Title"=w382:string)  [unwired: 4 in, 4 out]
                  n228 = call "CRYMessage Dialog.vi"("Window Title"=w382, "YesNoCancel"=T3."OK", "Message Content"=w383) -> ()  [unwired: 7 in, 2 out]
                }
                frame #1 {
                  w392 = 0 ("input 2")
                  n229 = Obtain Queue(name (unnamed)="CRYMAIN_ACTION" ("YAxisTitle"), element data type="" ("Action Type")) -> (queue out=w387:refnum<queue>)  [unwired: 3 in, 2 out]
                  n230 = Format Into String("FILE_EXIT" ("initial string"), "Menu" ("input 1"), w392, w392) -> (resulting string=w390:string)  [unwired: 3 in, 1 out]
                  n231 = Enqueue Element(queue=w387, element=w390) -> ()  [unwired: 1 in, 4 out]
                }
              }
            }
          }
        }
        frame "HELP_SHOW_CONTEXT" {
          n232 = disable-structure shown="Disabled" {
            frame Disabled {
              n233 = global read "CRYMainGlobal.vi" "Language"() -> (w397:T11)
              n234 = case shown="\"Korean\", \"Chinese traditional\"" w397 {
                frame "English", Default {
                  n235 = global read "CRYMain Sub Window Global.vi" "Main Menu Refnum"() -> (w400:refnum<k9>)
                  n236 = Get Menu Item Info(7:"HELP_SHOW_CONTEXT" ("item tag"), 11:w400) -> (4:w399:bool)  [unwired: 1 in, 6 out]
                  n237 = Not(x=w399) -> (.not. x?=w398:bool)
                  n238 = Control Help Window(1:w398) -> ()  [unwired: 1 out]
                }
                frame "Korean", "Chinese traditional" {
                  n239 = global read "CRYMainGlobal.vi" "top path"() -> (w403:path)
                  n240 = Build Path(base path=w403, name or relative path="Korean") -> (appended path=w402:path)
                  n241 = Build Path(base path=w402, name or relative path="InstallManual.pdf") -> (appended path=w406:path)
                  n242 = call "CRYOpen Manual.vi"("appended path"=w406) -> ()  [unwired: 11 out]
                }
              }
            }
            frame Enabled {
            }
          }
          n243 = global read "CRYMain Sub Window Global.vi" "Main Menu Refnum"() -> (w395:refnum<k9>)
          n244 = Get Menu Item Info(7:"HELP_SHOW_CONTEXT" ("item tag"), 11:w395) -> (4:w394:bool)  [unwired: 1 in, 6 out]
          n245 = Not(x=w394) -> (.not. x?=w393:bool)
          n246 = Control Help Window(1:w393) -> ()  [unwired: 1 out]
        }
        frame "HELP_COMPANYWEB" {
          n247 = disable-structure shown="Disabled" {
            frame Disabled {
              n248 = global read "CRYMainGlobal.vi" "Language"() -> (w408:T11)
              n249 = case shown="Default" w408 {
                frame Default {
                  n250 = call-poly <vilib>:"Open URL in Default Browser.vi"("URL"="http://www.crylab.com/Info/About.asp") -> ()  [unwired: 1 in, 6 out]
                }
                frame "Korean", "Chinese traditional" {
                  n251 = global read "CRYMainGlobal.vi" "top path"() -> (w411:path)
                  n252 = Build Path(base path=w411, name or relative path="Korean") -> (appended path=w410:path)
                  n253 = Build Path(base path=w410, name or relative path="DevHistory.mht") -> (appended path=w414:path)
                  n254 = call-poly <vilib>:"Open URL in Default Browser.vi"("path"=w414) -> ("error out"=w413:errorcluster)  [unwired: 1 in, 5 out]
                  n255 = case shown="No Error" w413 {
                    frame No Error {
                    }
                    frame Error {
                    }
                  }
                }
              }
            }
            frame Enabled {
            }
          }
          n256 = call-poly <vilib>:"Open URL in Default Browser.vi"("URL"="http://www.crysound.com") -> ()  [unwired: 1 in, 6 out]
        }
        frame "HELP_PRODUCTWEB" {
          n257 = disable-structure shown="Disabled" {
            frame Disabled {
              n258 = global read "CRYMainGlobal.vi" "Language"() -> (w417:T11)
              n259 = case shown="Default" w417 {
                frame Default {
                  n260 = call-poly <vilib>:"Open URL in Default Browser.vi"("URL"="http://www.crylab.com/Info/ProductUsedList.asp") -> ()  [unwired: 1 in, 6 out]
                }
                frame "Korean", "Chinese traditional" {
                  n261 = global read "CRYMainGlobal.vi" "top path"() -> (w421:path)
                  n262 = Build Path(base path=w421, name or relative path="ProductInfor.mht") -> (appended path=w420:path)
                  n263 = call-poly <vilib>:"Open URL in Default Browser.vi"("path"=w420) -> ("error out"=w419:errorcluster)  [unwired: 1 in, 5 out]
                  n264 = case shown="No Error" w419 {
                    frame No Error {
                    }
                    frame Error {
                    }
                  }
                }
              }
            }
            frame Enabled {
            }
          }
          n265 = call-poly <vilib>:"Open URL in Default Browser.vi"("URL"="http://www.crysound.com/product.php") -> ()  [unwired: 1 in, 6 out]
        }
        frame "HELP_ABOUT" {
          n266 = call "CRYAbout.vi"() -> ()  [unwired: 4 out]
        }
        frame "HELP_TUTORIAL" {
          n267 = global read "CRYMainGlobal.vi" "Language"() -> (w426:T11)
          n268 = case shown="\"Korean\"" w426 {
            tunnel: ["CRYHelp\\English" ("name or relative path") "CRYHelp\\Chinese" ("name or relative path") "CRYHelp\\Korean" ("name or relative path")] -> w423
            frame "English", Default {
            }
            frame "Chinese" {
            }
            frame "Korean" {
            }
          }
          n269 = global read "CRYMainGlobal.vi" "top path"() -> (w425:path)
          n270 = Build Path(base path=w425, name or relative path=w423) -> (appended path=w424:path)
          n271 = Build Path(base path=w424, name or relative path="CRY6181Tutor.pdf") -> (appended path=w427:path)
          n272 = call "CRYOpen Manual.vi"("appended path"=w427) -> ()  [unwired: 11 out]
        }
        frame "HELP_USER_MANUAL" {
          n273 = global read "CRYMainGlobal.vi" "Language"() -> (w433:T11)
          n274 = case shown="\"Korean\"" w433 {
            tunnel: ["CRYHelp\\English" ("name or relative path") "CRYHelp\\Chinese" ("name or relative path") "CRYHelp\\Korean" ("name or relative path")] -> w434
            frame "English", Default {
            }
            frame "Chinese" {
            }
            frame "Korean" {
            }
          }
          n275 = global read "CRYMainGlobal.vi" "top path"() -> (w435:path)
          n276 = Build Path(base path=w435, name or relative path=w434) -> (appended path=w432:path)
          n277 = Build Path(base path=w432, name or relative path="CRY6181Manual.pdf") -> (appended path=w436:path)
          n278 = call "CRYOpen Manual.vi"("appended path"=w436) -> ()  [unwired: 11 out]
        }
        frame "CRY_RECENTPROJECT_TAG0", "CRY_RECENTPROJECT_TAG1", "CRY_RECENTPROJECT_TAG2", "CRY_RECENTPROJECT_TAG3", "CRY_RECENTPROJECT_TAG4" {
          n279 = Match Pattern(string=w445, regular expression="_TAG") -> (after substring=w442:string)  [unwired: 1 in, 3 out]
          n280 = String Length(string=w442) -> (length=w443:i32)
          n281 = case shown="Default" w443 {
            tunnel: w442 -> [w452 _]
            tunnel: [w448 _] -> w441
            frame Default {
              n282 = global read "CRYMainGlobal.vi" "Recent Item Names"() -> (w451:string[][])
              n283 = Decimal String To Number(string=w452) -> (number=w446:i32)  [unwired: 2 in, 1 out]
              n284 = Index Array(array=w451, index (row)=0 ("disabled index (col)"), index (col)=w446) -> (element=w449:string)
              n285 = call "CRYMain Menu Process LIB LIB.vi"("sOption"=w449, "sAction"="OpenProject") -> ("sData_Out"=w448:string)  [unwired: 9 in]
            }
            frame 0 {
            }
          }
          n286 = local write "sData_Out"(w441) -> ()
        }
        frame "MSG_FROM_PRJECT" {
          n287 = Unbundle By Name(w453) -> ("EventName"=w457:string, "Arg1"=w456:string, "Arg1 2"=w455:string, "Arg1 3"=w454:string)
          n288 = case shown="\"OpenProjectFullPath\"" w457 {
            tunnel: w453 -> [_ w462 _ _]
            tunnel: w456 -> [_ _ w469 w489]
            tunnel: w455 -> [_ _ w470 w488]
            tunnel: w454 -> [_ _ w468 w487]
            frame "False", Default {
            }
            frame "OpenProjectFullPath" {
              n289 = Unbundle By Name(w462) -> ("Arg1"=w459:string)
              n290 = String To Path(string=w459) -> (path=w461:path)
              n291 = call <vilib>:"Check if File or Folder Exists.vi"("path"=w461) -> ("file or folder exists?"=w460:bool)  [unwired: 8 in, 2 out]
              n292 = case shown="True" w460 {
                tunnel: w459 -> [_ w465]
                tunnel: [_ w464] -> w458
                frame False {
                  (unwired) "?????" ("message")
                  n293 = One Button Dialog(message="File not exist.") -> ()  [unwired: 1 in, 1 out]
                }
                frame True {
                  n294 = call "CRYMain Menu Process LIB LIB.vi"("sOption"=w465, "sAction"="OpenProject") -> ("sData_Out"=w464:string)  [unwired: 9 in]
                }
              }
              n295 = local write "sData_Out"(w458) -> ()
            }
            frame "OpenStepView" {
              n296 = flat-sequence {
                tunnel: w470 -> [w477]
                tunnel: w469 -> [w474]
                tunnel: w468 -> [w472]
                tunnel: [w472] -> w467
                tunnel: w467 -> [w483]
                frame #0 {
                  (unwired) "Load" ("sData")
                  n297 = call "CRYConvert ASCII to Unicode.vi"("ASCII"=w474) -> ("Unicode"=w473:string)  [unwired: 4 in]
                  n298 = global read "CRYView Global.vi" "cBootDATAVIEW"() -> (w479:T4)
                  n299 = Bundle By Name(cluster=w479, "sAction"="AddStep" ("sData"), "sData"=w477, "nData"=0, "sQueueName"="ViewStep" ("sData"), "sType"=w473) -> (w478:T4)
                  n300 = global write "CRYView Global.vi" "cBootDATAVIEW"(w478) -> ()
                }
                frame #1 {
                  n301 = Concatenate Strings("StepView" ("Window Type"), "&#&" ("string"), w483) -> (w481:string)
                  n302 = call "CRYAPI WSYSTEM.vi"("sData"=w481, "sOption"="NOFOCUS", "sAction"="DOCK_TAB") -> ()  [unwired: 1 in, 8 out]
                  n303 = local write "sData_Out"("CANCEL" ("sData_Out")) -> ()
                }
              }
            }
            frame "ADD_DOC" {
              w491 = "H&H" ("string")
              n304 = Concatenate Strings(w489, w491, w488, w491, w487) -> (w490:string)
              n305 = flat-sequence {
                tunnel: [w497] -> w495
                tunnel: w490 -> [w496]
                tunnel: [w496] -> w494
                tunnel: w495 -> [w506]
                tunnel: w494 -> [w503]
                tunnel: [w502] -> w493
                tunnel: [w501] -> w492
                tunnel: w493 -> [w508]
                tunnel: w492 -> [w507]
                frame #0 {
                  n306 = call "CRYAPI WSYSTEM.vi"("sData"="Document" ("Window Type"), "sOption"="", "sAction"="DOCK_TAB") -> ("tFrame_Out"=w497:T8)  [unwired: 1 in, 7 out]
                }
                frame #1 {
                  n307 = Unbundle By Name(w506) -> ("pWVI"=w505:refnum<vi>)
                  n308 = invoke class="VI" method="Ctrl Val.Set"(reference=w505, "Control Name"="sInsertVIName", "Value"=w503) -> (reference out=w502:refnum<vi>, error out=w501:errorcluster)  [unwired: 2 in, 3 out]
                }
                frame #2 {
                  n309 = case shown="No Error" w507 {
                    tunnel: w508 -> [w512 _]
                    frame No Error {
                      n310 = call "CRYGet Boolean Reference.vi"("Label Name"="ADD_FRAME", "VI Refnum"=w512) -> ("Boolean Ref"=w510:refnum<vi>)  [unwired: 7 in, 2 out]
                      n311 = property class="Bool"(reference=w510, "Val(Sgnl)"=TRUE ("Visible")) -> ()  [unwired: 1 in, 2 out]
                    }
                    frame Error {
                    }
                  }
                }
              }
            }
          }
        }
        frame "MSG_ATTACH_VIEW" {
          n312 = disable-structure shown="Disabled" {
            disable-tunnel: w514 -> [w532 _]
            frame Disabled {
              n313 = call "CRYDataView Function LIB.vi"("sAction"="GetViewByID", "nData"=w532) -> ("cView_Out"=w530:T9)  [unwired: 7 in, 2 out]
              n314 = Unbundle By Name(w530) -> ("pVIRef"=w529:refnum<vi>)
              n315 = invoke class="VI" method="Ctrl Val.Get"(reference=w529, "Control Name"="pVIRefParent") -> ("Get Control Value Variant"=w527:variant)  [unwired: 2 in, 3 out]
              n316 = Variant To Data(type="pVIRef", Variant=w527) -> ()  [unwired: 1 in, 2 out]
            }
            frame Enabled {
            }
          }
          n317 = global read "CRYView Global.vi" "cBootVIEW"() -> (w522:T4)
          n318 = global read "CRYNew View Global.vi" "DataView_Global"() -> (w521:T12[])
          n319 = Unbundle By Name(w522) -> ()  [unwired: 1 out]
          n320 = call "CRYGet DataView Arrary Idx.vi"("DataView Idx In"=w514) -> ("DataView Arrary Idx out"=w513:i32)  [unwired: 10 in]
          n321 = Index Array(array=w521, index=w513) -> (element=w520:T12)
          n322 = Unbundle By Name(w520) -> ("Graph Main VIRef"=w516:refnum<vi>)
          n323 = invoke class="VI" method="Ctrl Val.Get"(reference=w516, "Control Name"="pVIRefParent") -> ("Get Control Value Variant"=w518:variant)  [unwired: 2 in, 3 out]
          n324 = Variant To Data(type="pVIRef 2", Variant=w518) -> (data=w515:refnum<vi>)  [unwired: 1 in, 1 out]
          n325 = call "CRYGet Boolean Reference.vi"("Label Name"="AttachView", "VI Refnum"=w515) -> ("Exist?"=w524:bool, "Boolean Ref"=w523:refnum<vi>)  [unwired: 7 in, 1 out]
          n326 = case shown="True" w524 {
            tunnel: w523 -> [_ w534]
            frame False {
            }
            frame True {
              n327 = property class="Bool"(reference=w534, "Val(Sgnl)"=FALSE) -> ()  [unwired: 1 in, 2 out]
            }
          }
        }
        frame "MSG_OPEN_PROJECT" {
          n328 = global read "CRYMainGlobal.vi" "Command line"() -> (w536:string)
          n329 = call "CRYMain Menu Process LIB LIB.vi"("sOption"=w536, "sAction"="OpenProject") -> ("sData_Out"=w535:string)  [unwired: 9 in]
          n330 = local write "sData_Out"(w535) -> ()
        }
        frame "MSG_STEP_RECOVERY" {
          n331 = flat-sequence {
            tunnel: [w543] -> w541
            tunnel: [w542] -> w540
            tunnel: [w551] -> w538
            tunnel: [w553] -> w539
            tunnel: w541 -> [w551]
            tunnel: w540 -> [w553]
            tunnel: w539 -> [w566]
            tunnel: w538 -> [w565]
            frame #0 {
              n332 = while {
                stop <- w547 stop-if-true
                n333 = global read "CRYMain Sub Window Global.vi" "sTaskWSYSTEM"() -> (w549:string)
                n334 = global read "CRYProject Editor Global.vi" "Project Exist?"() -> (w546:bool)
                n335 = String Length(string=w549) -> (length=w548:i32)
                n336 = Wait (ms)(milliseconds to wait=u32 10) -> ()  [unwired: 1 out]
                n337 = Equal To 0?(x=w548) -> (x = 0?=w545:bool)
                n338 = And(x=w545, y=w546) -> (x .and. y?=w547:bool)
              }
              n339 = global read "CRYStepSetup Global.vi" "cStep"() -> (w544:T13)
              n340 = Unbundle By Name(w544) -> ("sStepName"=w543:string, "nStepVINo"=w542:i32)
            }
            frame #1 {
              n341 = global read "CRYProject Editor Global.vi" "TS Array"() -> (w552:T6)
              n342 = Unbundle By Name(w552) -> ("Steps"=w554:T7[])
              n343 = for {
                tunnel: w554 -> [w560] mode=indexing
                tunnel: w553 -> [w556]
                i -> [w555]
                stop <- w557 stop-if-true
                n344 = Unbundle By Name(w560) -> ("No.VI"=w559:i32)
                n345 = Equal?(x=w559, y=w556) -> (x = y?=w558:bool)
                n346 = case shown="True" w558 {
                  selector: w558 -> [w563 w564]
                  tunnel: [w563 w564] -> w557
                  tunnel: w556 -> [w562 _]
                  tunnel: w555 -> [w561 _]
                  frame True {
                    n347 = global write "CRYProject Editor Global.vi" "SelectTreeStepNumber"(w561) -> ()
                    n348 = global write "CRYProject Editor Global.vi" "Step Setup VI No"(w562) -> ()
                  }
                  frame False {
                  }
                }
              }
            }
            frame #2 {
              n349 = call "CRYStepSetup MNG.vi"("sAction"="Insert" ("sData"), "nData"=w566, "sStepName"=w565) -> ()  [unwired: 7 in, 2 out]
            }
          }
        }
        frame "MSG_CLOSE_FRAME" {
          n350 = flat-sequence {
            tunnel: w568 -> [w570]
            tunnel: [w570] -> w569
            tunnel: w569 -> [w579]
            frame #0 {
              n351 = while {
                stop <- w573 stop-if-true
                n352 = global read "CRYMain Sub Window Global.vi" "sTaskWSYSTEM"() -> (w575:string)
                n353 = global read "CRYProject Editor Global.vi" "Project Exist?"() -> (w572:bool)
                n354 = String Length(string=w575) -> (length=w574:i32)
                n355 = Wait (ms)(milliseconds to wait=u32 10) -> ()  [unwired: 1 out]
                n356 = Equal To 0?(x=w574) -> (x = 0?=w571:bool)
                n357 = And(x=w571, y=w572) -> (x .and. y?=w573:bool)
              }
            }
            frame #1 {
              n358 = Number To Decimal String(number=w579) -> (decimal integer string=w578:string)  [unwired: 1 in]
              n359 = call "CRYAPI WSYSTEM.vi"("sData"=w578, "sAction"="CLOSE_FRAME") -> ()  [unwired: 6 in, 4 out]
            }
          }
        }
        frame "ONE_SELFTEST" {
          n360 = flat-sequence {
            frame #0 {
              n361 = call "CRYInitialize Menu State.vi"("sAction"="One Start", "Is Disable?"=TRUE) -> ()  [unwired: 10 out]
            }
            frame #1 {
              n362 = global read "CRYMainGlobal.vi" "Sequence path"() -> (w584:path)
              n363 = Build Path(base path=w584, name or relative path="One\\Self Test.cry") -> (appended path=w585:path)
              n364 = Path To String(path=w585) -> (string=w583:string)
              n365 = call "CRYMain Menu Process LIB LIB.vi"("sOption"=w583, "sAction"="OpenProject") -> ()  [unwired: 9 in, 1 out]
            }
            frame #2 {
              n366 = global read "CRYRef nums global.vi" "Run project VI ref"() -> (w588:refnum<vi>)
              n367 = invoke class="VI" method="Run VI"(reference=w588, "Wait until done"=FALSE ("Wait Until Done")) -> ()  [unwired: 3 in, 5 out]
            }
          }
        }
        frame "ONE_CALMIC" {
          n368 = flat-sequence {
            frame #0 {
              n369 = call "CRYProject Editor PIC Change State.vi"("bChangeState"=FALSE ("Change State")) -> ()  [unwired: 11 in]
              n370 = call "CRYInitialize Menu State.vi"("sAction"="One Start", "Is Disable?"=TRUE) -> ()  [unwired: 10 out]
            }
            frame #1 {
              n371 = global read "CRYMainGlobal.vi" "Sequence path"() -> (w594:path)
              n372 = Build Path(base path=w594, name or relative path="One\\Microphone Calibration.cry") -> (appended path=w595:path)
              n373 = Path To String(path=w595) -> (string=w593:string)
              n374 = call "CRYMain Menu Process LIB LIB.vi"("sOption"=w593, "sAction"="OpenProject") -> ()  [unwired: 9 in, 1 out]
            }
            frame #2 {
              n375 = call "CRYMicrophone Calibration by One.vi"() -> ()  [unwired: 12 in]
            }
          }
        }
        frame "ONE_SETUP" {
          n376 = flat-sequence {
            frame #0 {
              n377 = call "CRYProject Editor PIC Change State.vi"("bChangeState"=FALSE ("Change State")) -> ()  [unwired: 11 in]
              n378 = call "CRYInitialize Menu State.vi"("sAction"="One Start", "Is Disable?"=TRUE) -> ()  [unwired: 10 out]
            }
            frame #1 {
              n379 = global read "CRYMainGlobal.vi" "Sequence path"() -> (w602:path)
              n380 = Build Path(base path=w602, name or relative path="One\\Time Selective Response One.cry") -> (appended path=w603:path)
              n381 = Path To String(path=w603) -> (string=w600:string)
              n382 = call "CRYMain Menu Process LIB LIB.vi"("sOption"=w600, "sAction"="OpenProject") -> ()  [unwired: 9 in, 1 out]
            }
            frame #2 {
              n383 = call "CRYInitialize Menu State.vi"("sAction"="One Init", "Is Disable?"=TRUE) -> ()  [unwired: 10 in]
            }
            frame #3 {
              n384 = call "CRYGet Window Temp Reference.vi"("sWindowName"="Sequence Generator", "sAction"="OPEN_WINDOW") -> ("pVIRef_Out"=w607:refnum<vi>)  [unwired: 5 in, 4 out]
              n385 = invoke class="VI" method="FP.Open"(reference=w607, "Activate"=TRUE ("Activate?"), "State"=T2."Standard") -> ()  [unwired: 2 in, 5 out]
            }
          }
        }
      }
    }
    frame #2 {
      n386 = local read "sData_Out"() -> (w613:string)
      n387 = case shown="\"MSG_FROM_PRJECT\"" w614 {
        tunnel: w613 -> [_ w620 w622 w629]
        tunnel: w612 -> [_ _ _ w628]
        frame Default {
        }
        frame "FILE_CLOSE" {
          n388 = Equal?(x=w620, y="CLOSE" ("sAction")) -> (x = y?=w618:bool)
          n389 = Select(t="ProjectNew" ("sAction"), s=w618, f="ProjectOpen" ("sAction")) -> (s? t:f=w615:string)
          n390 = call "CRYMain Window Menu Setting.vi"("sAction"=w615) -> ()  [unwired: 11 out]
        }
        frame "CRY_RECENTPROJECT_TAG0", "CRY_RECENTPROJECT_TAG1", "CRY_RECENTPROJECT_TAG2", "CRY_RECENTPROJECT_TAG3", "CRY_RECENTPROJECT_TAG4", "FILE_NEW_PROJECT", "FILE_OPEN_PROJECT", "FILE_SAVE", "FILE_SAVE_AS", "MSG_OPEN_PROJECT" {
          n391 = case shown="\"CANCEL\"" w622 {
            tunnel: ["ProjectOpen" ("sAction") w624] -> w621
            frame Default {
            }
            frame "CANCEL" {
              n392 = global read "CRYProject Editor Global.vi" "Project Exist?"() -> (w627:bool)
              n393 = Select(t="ProjectOpen" ("sAction"), s=w627, f="ProjectNew" ("sAction")) -> (s? t:f=w624:string)
            }
          }
          n394 = call "CRYMain Window Menu Setting.vi"("sAction"=w621) -> ()  [unwired: 11 out]
        }
        frame "MSG_FROM_PRJECT" {
          n395 = case shown="True" w628 {
            tunnel: w629 -> [_ w631]
            frame False {
            }
            frame True {
              n396 = case shown="\"CANCEL\"" w631 {
                tunnel: ["ProjectOpen" ("sAction") w633] -> w630
                frame Default {
                }
                frame "CANCEL" {
                  n397 = global read "CRYProject Editor Global.vi" "Project Exist?"() -> (w636:bool)
                  n398 = Select(t="ProjectOpen" ("sAction"), s=w636, f="ProjectNew" ("sAction")) -> (s? t:f=w633:string)
                }
              }
              n399 = call "CRYMain Window Menu Setting.vi"("sAction"=w630) -> ()  [unwired: 11 out]
            }
          }
        }
      }
    }
    frame #3 {
      n400 = call "CRYProject Editor PIC Action End.vi"() -> ()  [unwired: 12 in]
    }
  }
